vi "Graph and chart difference_0.vi"() -> ()   [LabVIEW 2015]
panel:
  in  "Tab Control":enum32{"Page 1", "Page 2"}(tab)
  out "Waveform Graph":dbl[](graph)
  out "Waveform Chart":dbl(graph)
  in  "Save wave pic Invoke Node":path
  # "Using while loop plot data waveform chart in loop its plot every loop"
  # "Using while loop plot data waveform graph outside of loop its plot after loop complete"
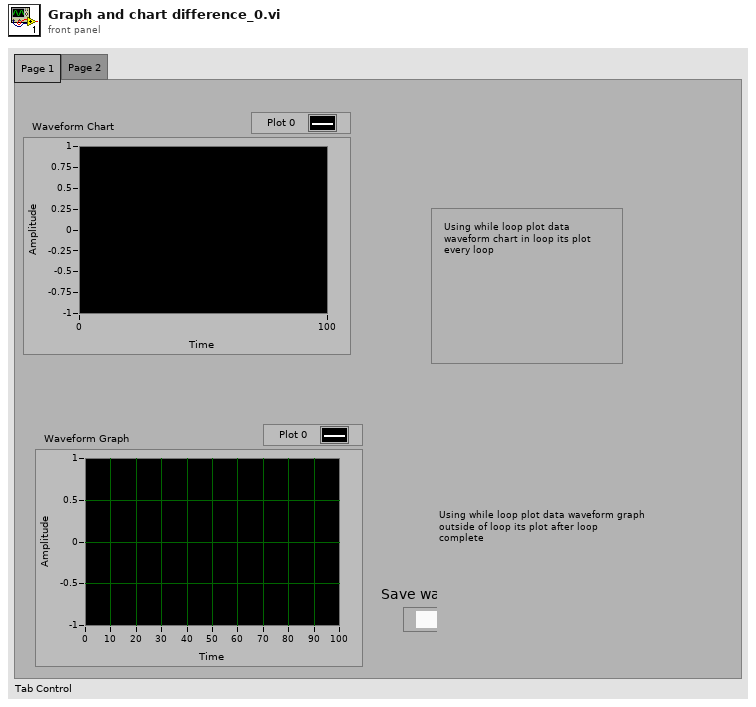
[diagram p1: front panel]
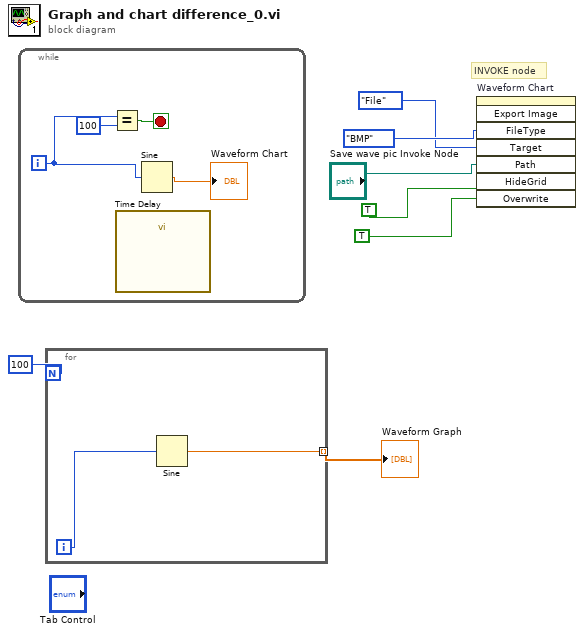
[diagram p0: block diagram]
diagram:
  # "INVOKE node"
  n1 = while {
    i -> [w10]
    stop <- w8 stop-if-true
    n2 = Equal?(x=w10, y=100) -> (x = y?=w8:bool)
    n3 = call "Time Delay"() -> ()  [unwired: 11 in, 1 out]
    n4 = Sine(x=w10) -> (sin(x)=→"Waveform Chart":dbl)
  }
  n5 = for {
    N: 100 -> [_]
    tunnel: [w12] -> w6 mode=indexing
    i -> [w13]
    n6 = Sine(x=w13) -> (sin(x)=w12:dbl)
  }
  "Waveform Graph" <- w6
  n7 = invoke on="Waveform Chart" class="WFChart (strict)" method="Export Image"("FileType"=enum32{"BMP", "EPS", "EMF", "PICT"}."BMP" ("File Type"), "Target"=enum32{"File", "Clipboard"}."File", "Path"="Save wave pic Invoke Node", "HideGrid"=TRUE ("Hide Grid"), "Overwrite"=TRUE ("Always Overwrite")) -> ()  [unwired: 3 in, 8 out]
